vi "AlliGator Remove Phasor Plot.vi"(8 "error in (no error)":errorcluster, 9 "Phasor Reference 1 Refnum":refnum<vi>, 10 "Selected Plot Info":T1, 11 "AlliGator IV DVR in":refnum<data-value>) -> (0 "error out":errorcluster, 2 "Message":string, 3 "AlliGator IV DVR out":refnum<data-value>)   [LabVIEW 2021, in "AlliGator Phasor Graph.lvlib"]
doc: "Removes Phasor Plot from Phasor Graph.\n\nNote that other actions need to be performed to remove the associated data and metadata."
uses:
  AlliGator Phasor Graph.lvlib
  Graphs/XY Graph/XY Graph Selected Plot Info.ctl
  Graphs/XY Graph/XY Graph Refnum.ctl
  <vilib>/Utility/miscctls.llb/LVPoint32TypeDef.ctl
  AlliGator Internal Variables v2.ctl
  <vilib>/vision/Image Controls.llb/IMAQ Image.ctl
  AlliGator Gate Image Set.ctl
  AlliGator FLI Dataset Type.ctl
  AlliGator Data Series Type.ctl
  AlliGator Dataset Channel.ctl
  AlliGator Gate Arithmetic.ctl
  AlliGator Displayed Image.ctl
  Image/Named ROI Description.ctl
  AlliGator Decay Metadata v3.ctl
  AlliGator Decay Background Subtraction Info.ctl
  AlliGator Baseline Subtraction Method.ctl
  Graphs/XY Graph/XY Graph Plot Shift Parameters.ctl
  Graphs/XY Graph/XY Graph Plot Shift Method.ctl
  AlliGator Decay Extrapolation Parameters.ctl
  Phasor/Calibration Phasor (m, phi).ctl
  Phasor/Phasor Reference Series.ctl
  Phasor/Phasor Calibration Map v2.ctl
  Phasor/Phasor (g, s).ctl
  AlliGator Raw Phasor Plot Data v4.ctl
  Phasor/Phasor Standard Deviation Options.ctl
  AlliGator Phasor Multi-Harmonic Data.ctl
  Phasor/Phasor Harmonic Data.ctl
  AlliGator Decay Fit Options & Parameters v2.ctl
  Fits/IRF(X)PSED/Decay Fit Options v2.ctl
  Fits/Decay Convolution/Decay Model.ctl
  Fits/Residual Type.ctl
  Fits/IRF(X)PSED/Fit Weights Type.ctl
  Fits/Non-linear Fitting Method v2.ctl
  Fits/Fit Calculation Method.ctl
  Fits/Non-linear Fitting Algorithm.ctl
  AlliGator Decay Fit Parameter Constraints 2.ctl
  Fits/IRF(X)PSED/Decay Fit Parameters In List.ctl
  Fits/IRF(X)PSED/MLE Baseline Offset Type.ctl
  AlliGator Decay Preprocessing Parameters.ctl
  Fits/IRF(X)PSED/Decay Fit Parameters & Derived Quantities List.ctl
  Graphs/XY Graph/XY Graph Add-Ons.lvlib
  AlliGator Phasor Calibration.lvlib
  AlliGator Source Image.lvlib
  Phasor/Phasor.lvlib
  Image/Image.lvlib
  AlliGator Decay Preprocessing.lvlib
  AlliGator Files.lvlib
  AlliGator Phasor Plot.lvlib
  Fits/Fits.lvlib
  AlliGator Decay Fit.lvlib
  AlliGator Decay Fit Parameter Map.lvlib
  AlliGator Settings.lvlib
  AlliGator Dual-Channel Datasets.lvlib
  AlliGator Internal Variables.lvlib
panel:
  # "see the AlliGator License on the block diagram (Ctrl+E or Window:Show Block Diagram)"
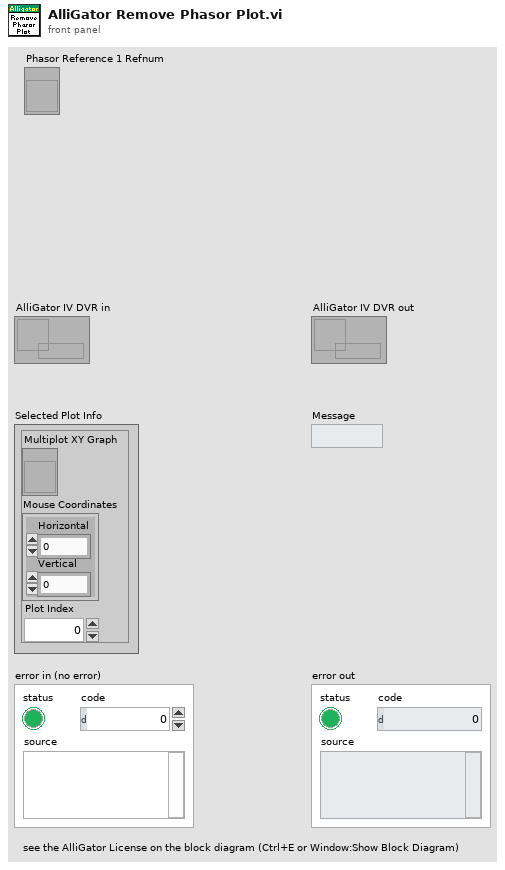
[diagram p1: front panel]
types:
  T1 = typedef "XY Graph Add-Ons.lvlib/XY Graph Selected Plot Info.ctl" = cluster{"Multiplot XY Graph":T2, "Mouse Coordinates":T3, "Plot Index":i32}
  T2 = typedef "XY Graph Add-Ons.lvlib/XY Graph Refnum.ctl" = refnum<vi>
  T3 = typedef "LVPoint32TypeDef.ctl" = cluster{"Horizontal":i32, "Vertical":i32}
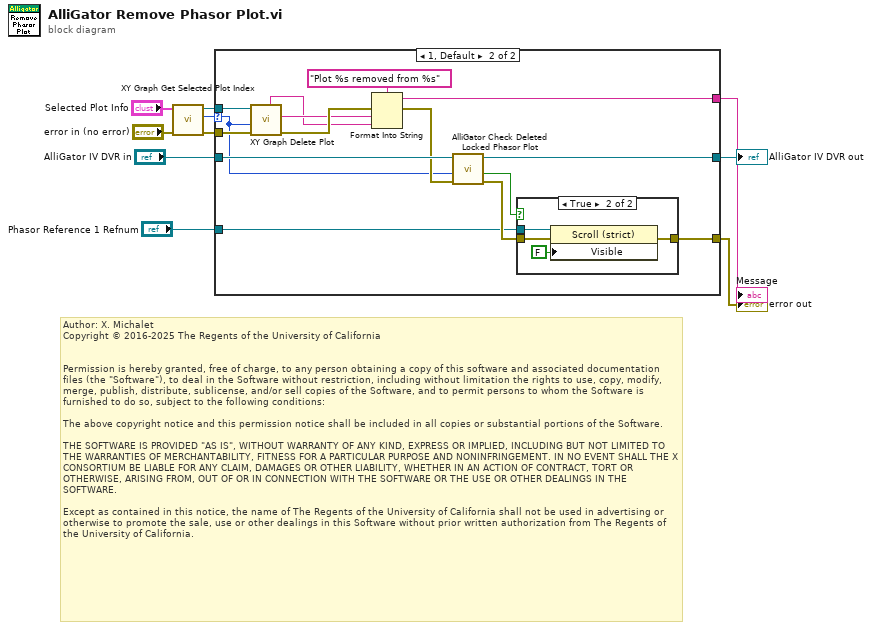
[diagram p0: block diagram]
diagram:
  # "Author: X. Michalet\nCopyright © 2016-2025 The Regents of the University of California\n \n\nPermission is hereby granted, free of charge, to any person obtaining a copy of this software and associated documentation files (the \"Software\"), to deal in the Software without restriction, including without limitation the rights to use, copy, modify, merge, publish, distribute, sublicense, and/or sell copies of the Software, and to permit persons to whom the Software is furnished to do so, subject to the following conditions:\n\nThe above copyright notice and this permission notice shall be included in all copies or substantial portions of the Software.\n\nTHE SOFTWARE IS PROVIDED \"AS IS\", WITHOUT WARRANTY OF ANY KIND, EXPRESS OR IMPLIED, INCLUDING BUT NOT LIMITED TO THE WARRANTIES OF MERCHANTABILITY, FITNESS FOR A PARTICULAR PURPOSE AND NONINFRINGEMENT. IN NO EVENT SHALL THE X CONSORTIUM BE LIABLE FOR ANY CLAIM, DAMAGES OR OTHER LIABILITY, WHETHER IN AN ACTION OF CONTRACT, TORT OR OTHERWISE, ARISING FROM, OUT OF OR IN CONNECTION WITH THE SOFTWARE OR THE USE OR OTHER DEALINGS IN THE SOFTWARE.\n\nExcept as contained in this notice, the name of The Regents of the University of California shall not be used in advertising or otherwise to promote the sale, use or other dealings in this Software without prior written authorization from The Regents of the University of California."
  n1 = call "XY Graph Get Selected Plot Index.vi"("error in (no error)"="error in (no error)", "Selected Plot Info"="Selected Plot Info") -> ("error out"=w8:errorcluster, "Plot at Coordinates"=w6:i32, "XYGraph out"=w7:T2)  [unwired: 6 in, 1 out]
  n2 = case shown="1, Default" w6 {
    selector: w6 -> [_ w17]
    tunnel: "AlliGator IV DVR in" -> [w12 w19]
    tunnel: [w12 w19] -> w2
    tunnel: w7 -> [_ w26]
    tunnel: w8 -> [w11 w25]
    tunnel: [w11 w14] -> w9
    tunnel: [_ w21] -> w10
    tunnel: "Phasor Reference 1 Refnum" -> [_ w13]
    frame -1, 0 {
    }
    frame 1, Default {
      n3 = call "XY Graph Delete Plot.vi"("Error In"=w25, "Plot Index"=w17, "XYGraph Ref"=w26) -> ("Error Out"=w24:errorcluster, "Plot Name"=w23:string, "Graph Caption (or Label)"=w22:string)  [unwired: 5 in, 1 out]
      n4 = Format Into String(format string="Plot %s removed from %s", error in=w24, w23, w22) -> (resulting string=w21:string, error out=w18:errorcluster)  [unwired: 1 in]
      n5 = call "AlliGator Check Deleted Locked Phasor Plot.vi"("Error In"=w18, "Deleted Plot Index"=w17, "AlliGator Internal Variables DVR"=w19) -> ("Error Out"=w15:errorcluster, "Hide Reference 1 Control"=w16:bool)  [unwired: 6 in, 1 out]
      n6 = case shown="True" w16 {
        tunnel: w13 -> [_ w31]
        tunnel: w15 -> [w27 w30]
        tunnel: [w27 w29] -> w14
        frame False {
        }
        frame True {
          n7 = property class="Scroll (strict)"(reference=w31, error in=w30, "Visible"=FALSE) -> (error out=w29:errorcluster)  [unwired: 1 out]
        }
      }
    }
  }
  "Message" <- w10
  "error out" <- w9
  "AlliGator IV DVR out" <- w2
